vi "Configure Lockin.vi"(8 "error in (no error)":errorcluster, 10 "IV Run":T1={"Pattern"=enum."Ramp /\\", "Cycles"=0.0, "Rate"=1.0, "End"=1.0, "Start"=1.0}, 11 "MeasurementSMO in":refnum<class "AFM_Litho_Plugin.IV.lvclass">) -> (0 "error out":errorcluster, 3 "MeasurementSMO out":refnum<class "AFM_Litho_Plugin.IV.lvclass">)   [LabVIEW 2019, in "AFM_Litho_Plugin.IV.lvclass"]
uses:
  AFM_Litho_Plugin.IV.lvclass
  Typedefs/PrivateEvents--AFM_Litho_Plugin.IV.IV Run--Local.ctl
  AFM_Litho_Plugin.IV.lvclass/AFM_Litho_Plugin.IV.ctl
  <userlib>/LevyLab/Lockin-Multichannel/Instrument.DAQ/Typedefs/Sweep.Configuration--Cluster.ctl
  <userlib>/LevyLab/Lockin-Multichannel/Instrument.DAQ/Typedefs/Sweep.Channel--Cluster--Array.ctl
  <userlib>/LevyLab/Lockin-Multichannel/Instrument.DAQ/Typedefs/Sweep.Channel--Cluster.ctl
  <userlib>/LevyLab/Lockin-Multichannel/Instrument.DAQ/Typedefs/Sweep.Pattern--Enum.ctl
  a20de67c-2847-421e-9fbf-426d54e316b7.vi
  a20de67c-2847-421e-9fbf-426d54e316b7.vi/ff40df25-0e41-4205-825d-56c19dc320b6.vi
  <vilib>/Utility/Debug Log/Display.vi
  <vilib>/addons/_JKI.lib/Serialization/JSON/JKI JSON Serialization.lvlib
  <userlib>/LevyLab/Lockin-Multichannel/Instrument.DAQ/Instrument.DAQ.lvclass
  <userlib>/LevyLab/Lockin-Multichannel/Instrument.Lockin/Instrument.Lockin.lvclass
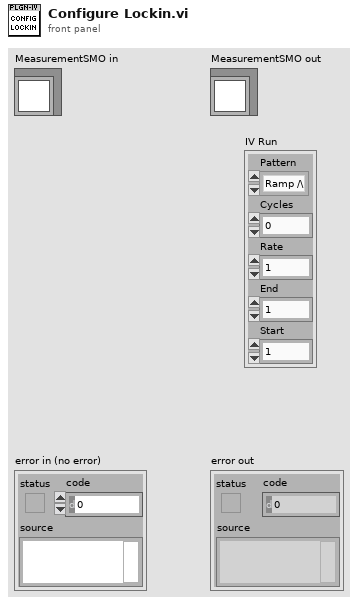
[diagram p1: front panel]
types:
  T1 = typedef "AFM_Litho_Plugin.IV.lvclass/PrivateEvents--AFM_Litho_Plugin.IV.IV Run--Local.ctl" = cluster{"Pattern":enum16{"Ramp /", "Ramp /\\", "Smooth Ramp _/", "Smooth Ramp _/\\_", "Frequency"}, "Cycles":dbl, "Rate":dbl, "End":dbl, "Start":dbl}
  T2 = typedef "Instrument.DAQ.lvclass/Sweep.Channel--Cluster.ctl" = cluster{"Enable?":bool, "Channel":u16, "Start":dbl, "End":dbl, "Pattern":T3}
  T3 = typedef "Instrument.DAQ.lvclass/Sweep.Pattern--Enum.ctl" = enum16{"Ramp /", "Ramp /\\", "Smooth Ramp _/", "Smooth Ramp _/\\_", "Frequency"}
  T4 = typedef "Instrument.DAQ.lvclass/Sweep.Configuration--Cluster.ctl" = cluster{"Sweep Time (s)":dbl, "Initial Wait (s)":dbl, "Return to Start":bool, "Channels":T5}
  T5 = typedef "Instrument.DAQ.lvclass/Sweep.Channel--Cluster--Array.ctl" = T2[]
  T6 = enum16{"Ramp /", "Ramp /\\", "Smooth Ramp _/", "Smooth Ramp _/\\_", "Frequency"}
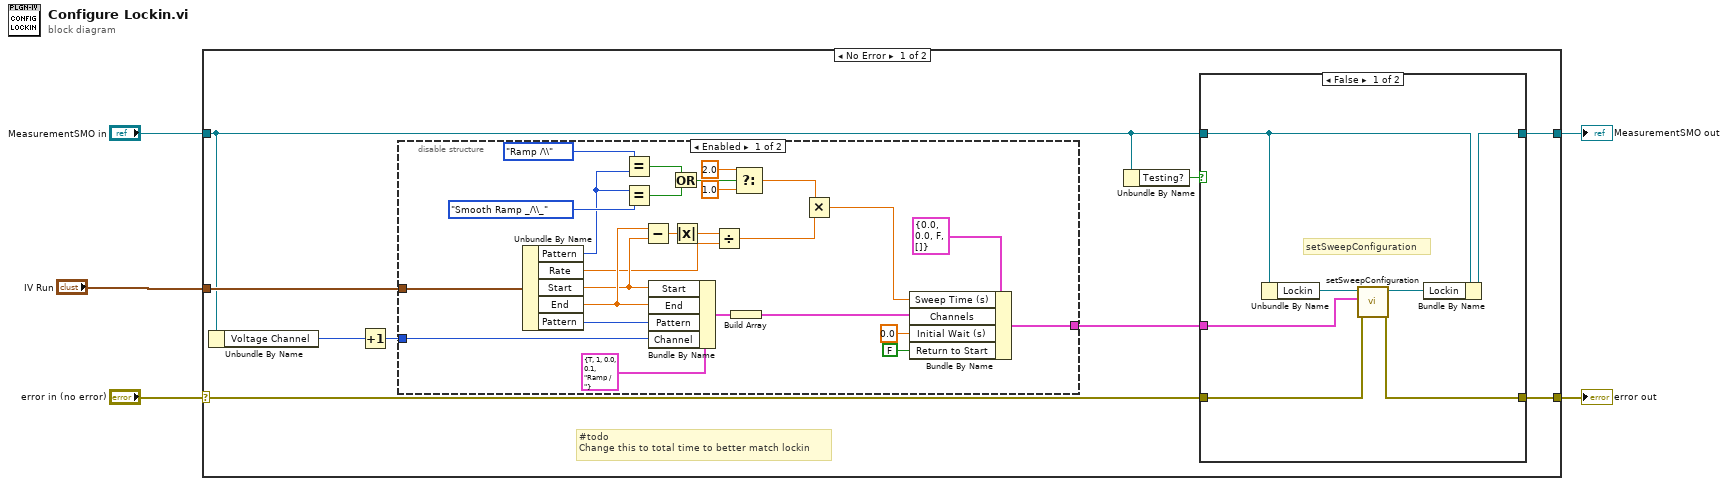
[diagram p0: block diagram]
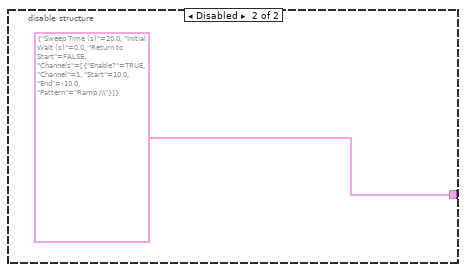
[diagram p2: hidden frame]
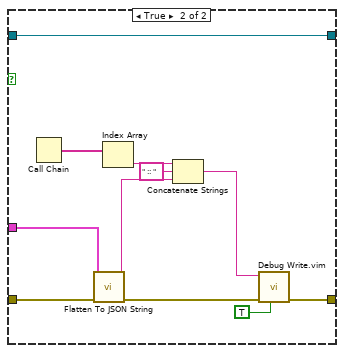
[diagram p3: hidden frame]
diagram:
  n1 = case shown="No Error" "error in (no error)" {
    selector: "error in (no error)" -> [w13 w61]
    tunnel: [w14 w61] -> w4
    tunnel: [w12 w60] -> w2
    tunnel: "MeasurementSMO in" -> [w8 w60]
    tunnel: "IV Run" -> [w11 _]
    frame No Error {
      # "#todo\nChange this to total time to better match lockin"
      n2 = Unbundle By Name(w8) -> ("Voltage Channel"=w7:u16)
      n3 = Increment(x=w7) -> (x+1=w6:u16)
      n4 = disable-structure shown="Enabled" {
        disable-tunnel: w11 -> [w40 _]
        disable-tunnel: [w29 T4 {"Sweep Time (s)"=20.0, "Initial Wait (s)"=0.0, "Return to Start"=FALSE, "Channels"=[{"Enable?"=TRUE, "Channel"=1, "Start"=10.0, "End"=-10.0, "Pattern"=enum."Ramp /\\"}]} ("Configure Sweep")] -> w10
        disable-tunnel: w6 -> [w17 _]
        frame Enabled {
          n5 = Unbundle By Name(w40) -> ("Pattern"=w25:T6, "Rate"=w30:dbl, "Start"=w33:dbl, "End"=w34:dbl, "Pattern"=w38:T6)
          n6 = Equal?(x=T6."Ramp /\\" ("Pattern"), y=w25) -> (x = y?=w28:bool)
          n7 = Equal?(x=w25, y=T6."Smooth Ramp _/\\_" ("Pattern")) -> (x = y?=w18:bool)
          n8 = Subtract(x=w34, y=w33) -> (x-y=w32:dbl)
          n9 = Bundle By Name(cluster=T2 {"Enable?"=TRUE, "Channel"=1, "Start"=0.0, "End"=0.1, "Pattern"=enum."Ramp /"} ("Sweep"), "Start"=w33, "End"=w34, "Pattern"=w38, "Channel"=w17) -> (w37:T2)
          n10 = Or(x=w28, y=w18) -> (x .or. y?=w24:bool)
          n11 = Absolute Value(x=w32) -> (abs(x)=w31:dbl)
          n12 = Divide(x=w31, y=w30) -> (x/y=w20:dbl)
          n13 = Build Array(w37) -> (w39:T2[])
          n14 = Select(t=2.0, s=w24, f=1.0) -> (s? t:f=w21:dbl)
          n15 = Multiply(x=w21, y=w20) -> (x*y=w19:dbl)
          n16 = Bundle By Name(cluster=T4 {"Sweep Time (s)"=0.0, "Initial Wait (s)"=0.0, "Return to Start"=FALSE, "Channels"=[]} ("Configure Sweep"), "Sweep Time (s)"=w19, "Channels"=w39, "Initial Wait (s)"=0.0, "Return to Start"=FALSE) -> (w29:T4)
        }
        frame Disabled {
        }
      }
      n17 = Unbundle By Name(w8) -> ("Testing?"=w9:bool)
      n18 = case shown="False" w9 {
        tunnel: [w42 w54] -> w14
        tunnel: w13 -> [w43 w56]
        tunnel: [w48 w59] -> w12
        tunnel: w8 -> [w47 w59]
        tunnel: w10 -> [w44 w49]
        frame False {
          # "setSweepConfiguration"
          n19 = Unbundle By Name(w47) -> ("Lockin"=w46:refnum<class "Instrument.Lockin.lvclass">)
          n20 = call <userlib>:"setSweepConfiguration.vi"("error in (no error)"=w43, "Configure Sweep"=w44, "Instrument.Lockin in"=w46) -> ("error out"=w42:errorcluster, "Instrument.Lockin out"=w45:refnum<class "Instrument.Lockin.lvclass">)  [unwired: 7 in]
          n21 = Bundle By Name(cluster=w47, "Lockin"=w45) -> (w48:refnum<class "AFM_Litho_Plugin.IV.lvclass">)
        }
        frame True {
          n22 = Call Chain() -> (call chain=w58:string[])
          n23 = call <vilib>:"Flatten To JSON String.vi"("error in (no error)"=w56, "Variant"=w49) -> ("error out"=w55:errorcluster, "JSON String"=w52:string)  [unwired: 8 in]
          n24 = Index Array(array=w58) -> (element=w57:string)  [unwired: 1 in]
          n25 = Concatenate Strings(w57, " :: " ("string"), w52) -> (w51:string)
          n26 = call "Debug Write.vim"("include timestamp? (F)"=TRUE, "error in (no error)"=w55, "value"=w51) -> ("error out"=w54:errorcluster)  [unwired: 8 in]
        }
      }
    }
    frame Error {
    }
  }
  "error out" <- w4
  "MeasurementSMO out" <- w2
